vi "Notifier Wait.vi"(8 "error in (no error)":errorcluster, 11 "Messaging in":refnum<class "Messaging.lvclass">) -> (0 "error out":errorcluster, 1 "Data":variant, 2 "Message":string, 3 "Messaging out":refnum<class "Messaging.lvclass">)   [LabVIEW 2023, in "Messaging.lvclass"]
uses:
  Messaging.lvclass
  Messaging.lvclass/Messaging.ctl
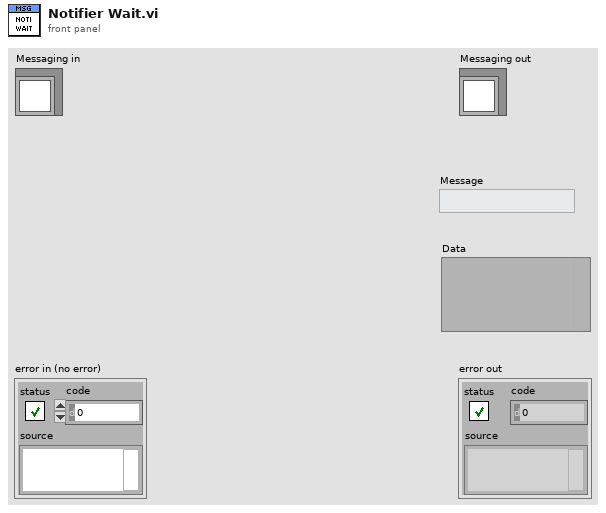
[diagram p1: front panel]
types:
  T1 = typedef "Msg.Noti.Ref.ctl" = refnum<notifier>
  T2 = typedef "Msg.Data.ctl" = cluster{"Message":string, "Data":variant}
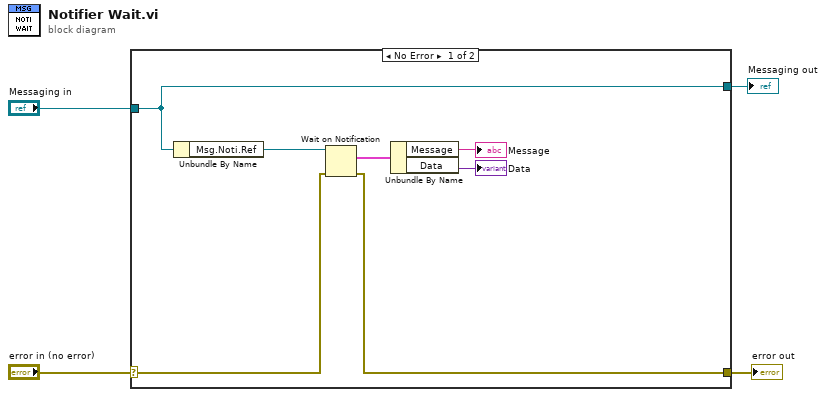
[diagram p0: block diagram]
diagram:
  n1 = case shown="No Error" "error in (no error)" {
    selector: "error in (no error)" -> [w10 w13]
    tunnel: [w5 w13] -> w3
    tunnel: [w6 w12] -> w1
    tunnel: "Messaging in" -> [w6 w12]
    frame No Error {
      n2 = Unbundle By Name(w6) -> ("Msg.Noti.Ref"=w11:T1)
      n3 = Wait on Notification(notifier=w11, error in (no error)=w10) -> (notification=w9:T2, error out=w5:errorcluster)  [unwired: 2 in, 2 out]
      n4 = Unbundle By Name(w9) -> ("Message"=→"Message":string, "Data"=→"Data":variant)
    }
    frame Error {
    }
  }
  "error out" <- w3
  "Messaging out" <- w1
